vi "in_create mesh grid (2D) (x array).vi"(11 "domain":dbl[](array[numeric])) -> (0 "error":i32, 2 "Y":dbl[][](array[numeric]), 3 "X":dbl[][](array[numeric]))   [LabVIEW 2017, in "NI_Gmath.lvlib"]
uses:
  <vilib>/gmath/NI_Gmath.lvlib
panel:
  # "Create Mesh Grid (2D)"
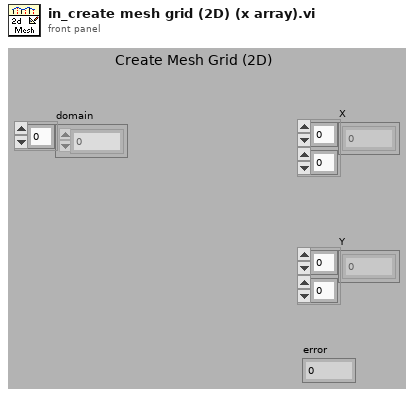
[diagram p1: front panel]
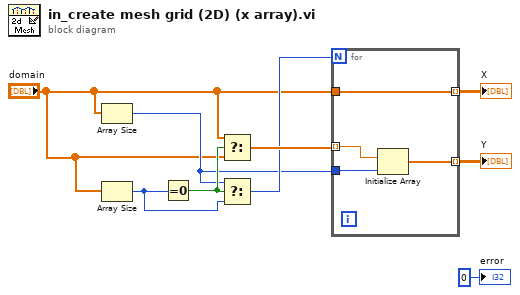
[diagram p0: block diagram]
diagram:
  n1 = Array Size(array="domain") -> (size(s)=w3:i32)
  n2 = Array Size(array="domain") -> (size(s)=w5:i32)
  n3 = Equal To 0?(x=w5) -> (x = 0?=w7:bool)
  n4 = Select(t="domain", s=w7, f="domain") -> (s? t:f=w6:dbl[])
  n5 = Select(t=w3, s=w7, f=w5) -> (s? t:f=w4:i32)
  n6 = for {
    N: w4 -> [_]
    tunnel: "domain" -> [w13]
    tunnel: [w13] -> w9 mode=indexing
    tunnel: w6 -> [w12] mode=indexing
    tunnel: [w11] -> w8 mode=indexing
    tunnel: w3 -> [w10]
    n7 = Initialize Array(w12, w10) -> (w11:dbl[])
  }
  "X" <- w9
  "Y" <- w8
  "error" <- 0 ("error")
